vi "CRC_Modbus.vi"(11 "字符串":string) -> (3 "输出变量":u16 format="%x")   [LabVIEW 2013]
panel:
  out "长度":i32
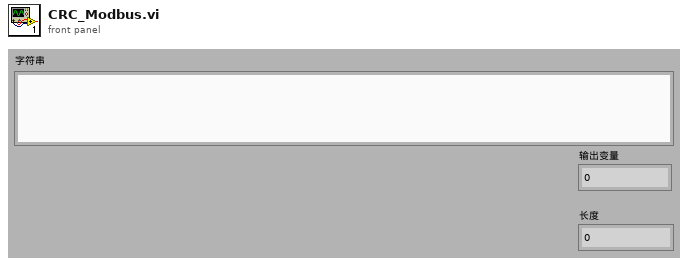
[diagram p1: front panel]
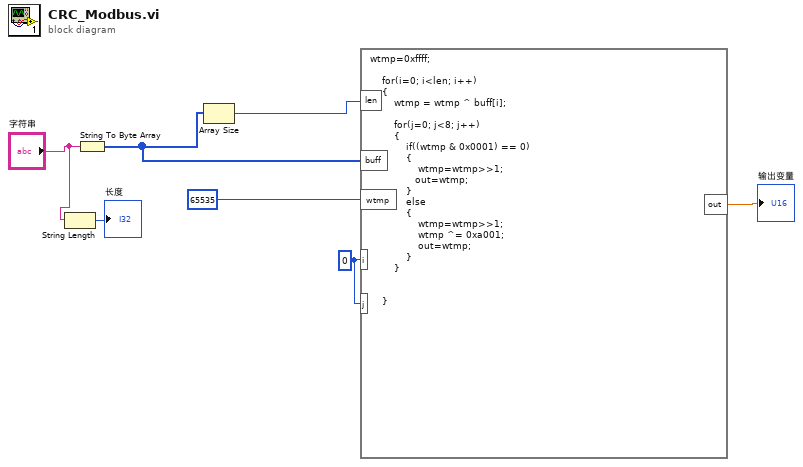
[diagram p0: block diagram]
diagram:
  w6 = u8 0 ("输入变量")
  n1 = String Length(string="字符串") -> (length=→"长度":i32)
  n2 = String To Byte Array(string="字符串") -> (unsigned byte array=w4:u8[])
  n3 = Array Size(array=w4) -> (size(s)=w1:i32)
  n4 = formula code="wtmp=0xffff;\n\n    for(i=0; i<len; i++) \n    {\n        wtmp = wtmp ^ buff[i];\n        \n        for(j=0; j<8; j++) \n        {\n            if((wtmp & 0x0001) == 0)\n            {\n                wtmp=wtmp>>1;  \n               out=wtmp;\n            } \n            else\n            {\n                wtmp=wtmp>>1;\n                wtmp ^= 0xa001;   \n                out=wtmp;\n            }\n        }\n        \n        \n    }"("buff"=w4, "wtmp"=u16 65535 ("数值"), "i"=w6, "j"=w6, "len"=w1) -> ("out"=→"输出变量":dbl)
